vi "Trilateration.vi"(8 "direction":bool) -> (1 "new point z":dbl=0.11811869208701314, 2 "new point y":dbl=0.8159406539564933, 3 "new point x":dbl=0.4340593460435067)   [LabVIEW 2018]
doc: "Calculates position of a point in 3D space which is at known distances from three points."
uses:
  <vilib>/measure/NI_MAPro.lvlib
  <vilib>/measure/matone.llb/Extract Multiple Tone Information 1 Chan.vi
  <vilib>/Analysis/NI_AALBase.lvlib
  <vilib>/Analysis/3filter.llb/Butterworth Filter (DBL).vi
  <vilib>/Analysis/3filter.llb/Filter Passband Type.ctl
  <resource>/objmgr/daqmx.rc
  <vilib>/DAQmx/read.llb/DAQmx Read (Analog 2D DBL NChan NSamp).vi
  <vilib>/DAQmx/configure/timing.llb/DAQmx Timing (Sample Clock).vi
  <vilib>/DAQmx/create/channels.llb/DAQmx Create Channel (AI-Voltage-Basic).vi
  <vilib>/DAQmx/configure/trigger.llb/DAQmx Start Trigger (None).vi
panel:
  in  "physical channels":tag="Dev2/ai0:1"
  in  "Sampling rate":dbl=10000.0 format="%0.2f"
  in  "stop":bool
  out "Waveform Graph":dbl[][](graph)
  in  "Change":bool
  in  "sampling freq: fs":dbl=1.0 format="%0.2f"
  in  "z 3":dbl
  in  "y 3":dbl
  in  "x 3":dbl=1.0
  in  "z 2":dbl
  in  "y 2":dbl
  in  "x 2":dbl=1.0
  in  "z":dbl
  in  "y":dbl
  in  "x":dbl=1.0
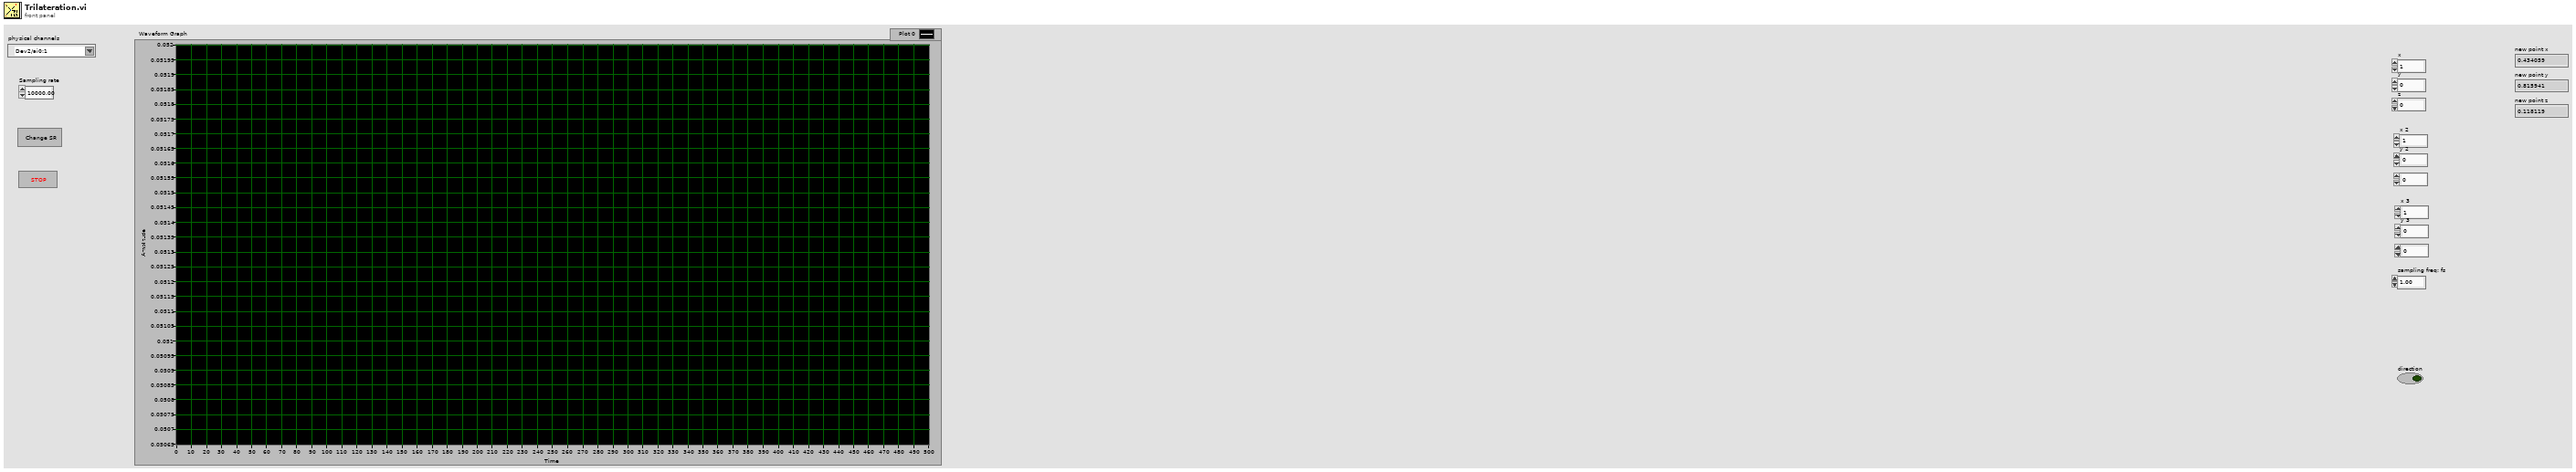
[diagram p1: front panel]
types:
  T1 = typedef "NI_AALBase.lvlib/Filter Passband Type.ctl" = enum32{"Lowpass", "Highpass", "Bandpass", "Bandstop"}
  T2 = cluster{"detected frequency":dbl, "detected amplitude":dbl, "detected phase (deg)":dbl}[]
  T3 = cluster{"[0]":cluster{"detected frequency":dbl, "detected amplitude":dbl, "detected phase (deg)":dbl}, "[1]":cluster{"detected frequency":dbl, "detected amplitude":dbl, "detected phase (deg)":dbl}, "[2]":cluster{"detected frequency":dbl, "detected amplitude":dbl, "detected phase (deg)":dbl}, "[3]":cluster{"detected frequency":dbl, "detected amplitude":dbl, "detected phase (deg)":dbl}, "[4]":cluster{"detected frequency":dbl, "detected amplitude":dbl, "detected phase (deg)":dbl}, "[5]":cluster{"detected frequency":dbl, "detected amplitude":dbl, "detected phase (deg)":dbl}, "[6]":cluster{"detected frequency":dbl, "detected amplitude":dbl, "detected phase (deg)":dbl}, "[7]":cluster{"detected frequency":dbl, "detected amplitude":dbl, "detected phase (deg)":dbl}, "[8]":cluster{"detected frequency":dbl, "detected amplitude":dbl, "detected phase (deg)":dbl}}
  T4 = cluster{"detected frequency":dbl, "detected amplitude":dbl, "detected phase (deg)":dbl}
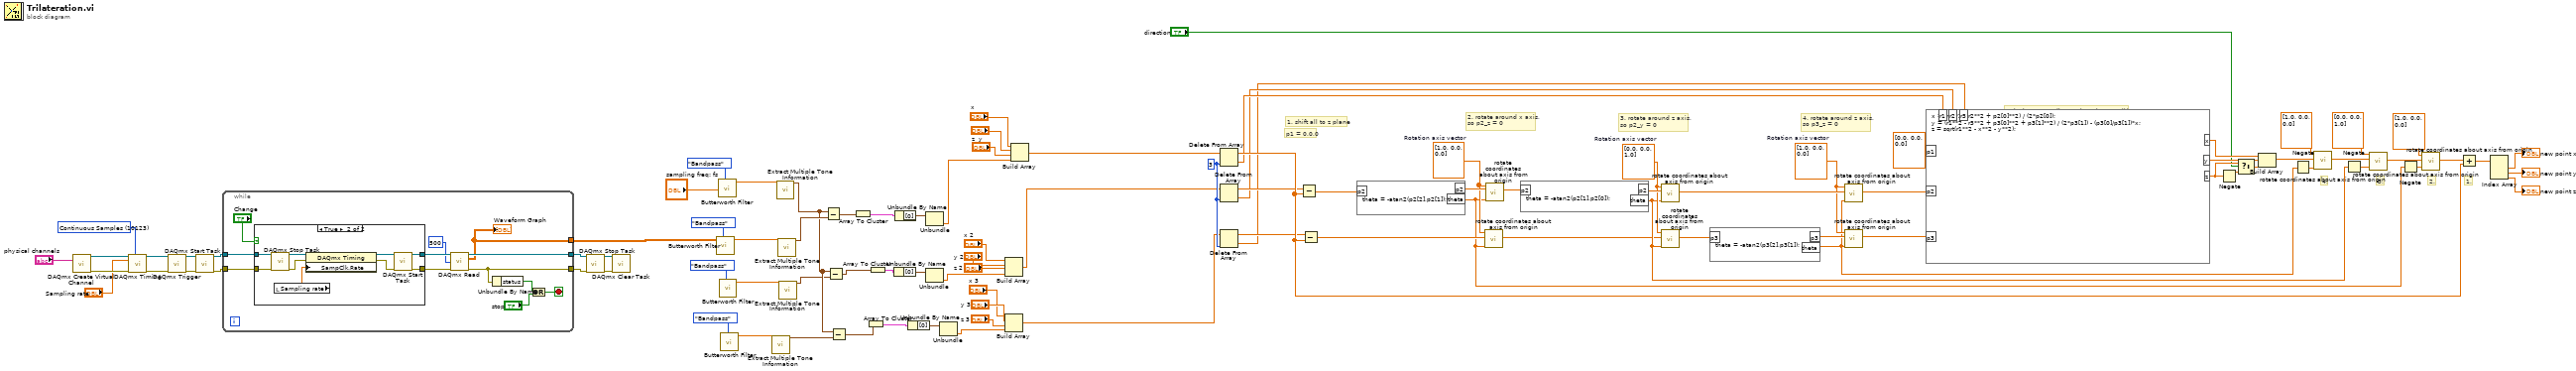
[diagram p0: block diagram]
diagram:
  w9 = 10123 items=["Finite Samples"=10178, "Continuous Samples"=10123, "Hardware Timed Single Point"=12522] ("sample mode")
  w65 = 3 ("index")
  w77 = dbl[] [1.0, 0.0, 0.0]  # Rotation axis vector
  w85 = dbl[] [1.0, 0.0, 0.0]  # Rotation axis vector
  w97 = dbl[] [0.0, 0.0, 1.0]  # Rotation axis vector
  # "1."
  # "2."
  # "3."
  # "4."
  # "Calculate, according to the rules on wiki"
  # "4. rotate around z axis,\nso p3_z = 0"
  # "2. rotate around x axis,\nso p2_z = 0"
  # "1. shift all to z plane"
  # "3. rotate around z axis,\nso p2_y = 0"
  # "p1 = 0,0,0"
  n1 = call-poly <vilib>:"DAQmx Create Virtual Channel.vi"("physical channels"="physical channels") -> ("task out"=w14:refnum<k21>, "error out"=w12:errorcluster)  [unwired: 13 in]
  n2 = call-poly <vilib>:"DAQmx Timing.vi"("task/channels in"=w14, "sample mode"=w9, "rate"="Sampling rate", "error in"=w12) -> ("task out"=w5:refnum<k21>, "error out"=w3:errorcluster)  [unwired: 10 in]
  n3 = call-poly <vilib>:"DAQmx Trigger.vi"("task/channels in"=w5, "error in"=w3) -> ("task out"=w4:refnum<k21>, "error out"=w2:errorcluster)  [unwired: 12 in]
  n4 = call <vilib>:"DAQmx Start Task.vi"("task/channels in"=w4, "error in"=w2) -> ("task out"=w7:refnum<k21>, "error out"=w8:errorcluster)  [unwired: 12 in]
  n5 = while {
    tunnel: w7 -> [w105]
    tunnel: [w110] -> w13
    tunnel: w8 -> [w103]
    tunnel: [w108] -> w11
    tunnel: [w99] -> w1
    stop <- w109 stop-if-true
    n6 = case shown="True" "Change" {
      tunnel: w105 -> [w112 w120]
      tunnel: [w112 w115] -> w104
      tunnel: w103 -> [w111 w119]
      tunnel: [w111 w113] -> w102
      frame False {
      }
      frame True {
        n7 = call <vilib>:"DAQmx Stop Task.vi"("task/channels in"=w120, "error in"=w119) -> ("task out"=w118:refnum<k21>, "error out"=w117:errorcluster)  [unwired: 12 in]
        n8 = local read "Sampling rate"() -> (w121:dbl)
        n9 = property class="DAQmx Timing"(reference=w118, error in=w117, "SampClk.Rate"=w121) -> (reference out=w116:refnum<k21>, error out=w114:errorcluster)
        n10 = call <vilib>:"DAQmx Start Task.vi"("task/channels in"=w116, "error in"=w114) -> ("task out"=w115:refnum<k21>, "error out"=w113:errorcluster)  [unwired: 12 in]
      }
    }
    n11 = call-poly <vilib>:"DAQmx Read.vi"("task/channels in"=w104, "number of samples per channel"=500, "error in"=w102) -> ("task out"=w110:refnum<k21>, "data"=w99:dbl[][], "error out"=w108:errorcluster)  [unwired: 10 in]
    "Waveform Graph" <- w99
    n12 = Unbundle By Name(w108) -> ("status"=w107:bool)
    n13 = Or(x=w107, y="stop") -> (x .or. y?=w109:bool)
  }
  n14 = call <vilib>:"DAQmx Stop Task.vi"("task/channels in"=w13, "error in"=w11) -> ("task out"=w16:refnum<k21>, "error out"=w15:errorcluster)  [unwired: 12 in]
  n15 = call <vilib>:"DAQmx Clear Task.vi"("task in"=w16, "error in"=w15) -> ()  [unwired: 13 in, 1 out]
  n16 = call-poly <vilib>:"Butterworth Filter.vi"("filter type"=Filter_Passband_Type."Bandpass", "X"=w1) -> ("Filtered X"=w44:dbl[])  [unwired: 6 in, 1 out]
  n17 = call-poly <vilib>:"Butterworth Filter.vi"("filter type"=Filter_Passband_Type."Bandpass", "sampling freq: fs"="sampling freq: fs") -> ("Filtered X"=w45:dbl[])  [unwired: 6 in, 1 out]
  n18 = call-poly <vilib>:"Butterworth Filter.vi"("filter type"=Filter_Passband_Type."Bandpass") -> ("Filtered X"=w43:dbl[])  [unwired: 7 in, 1 out]
  n19 = call-poly <vilib>:"Butterworth Filter.vi"("filter type"=Filter_Passband_Type."Bandpass") -> ("Filtered X"=w42:dbl[])  [unwired: 7 in, 1 out]
  n20 = call-poly <vilib>:"Extract Multiple Tone Information.vi"("time signal in"=w42) -> ("multiple tone information"=w51:T2)  [unwired: 12 in, 2 out]
  n21 = call-poly <vilib>:"Extract Multiple Tone Information.vi"("time signal in"=w45) -> ("multiple tone information"=w52:T2)  [unwired: 12 in, 2 out]
  n22 = call-poly <vilib>:"Extract Multiple Tone Information.vi"("time signal in"=w44) -> ("multiple tone information"=w53:T2)  [unwired: 12 in, 2 out]
  n23 = call-poly <vilib>:"Extract Multiple Tone Information.vi"("time signal in"=w43) -> ("multiple tone information"=w50:T2)  [unwired: 12 in, 2 out]
  n24 = Subtract(x=w52, y=w53) -> (x-y=w40:T2)
  n25 = Subtract(x=w52, y=w50) -> (x-y=w31:T2)
  n26 = Subtract(x=w52, y=w51) -> (x-y=w32:T2)
  n27 = Array To Cluster(array=w40) -> (cluster=w39:T3)
  n28 = Array To Cluster(array=w32) -> (cluster=w34:T3)
  n29 = Array To Cluster(array=w31) -> (cluster=w36:T3)
  n30 = Unbundle By Name(w36) -> ("[0]"=w35:T4)
  n31 = Unbundle By Name(w39) -> ("[0]"=w38:T4)
  n32 = Unbundle By Name(w34) -> ("[0]"=w33:T4)
  n33 = Unbundle(w35) -> ("detected phase (deg)"=w30:dbl)  [unwired: 2 out]
  n34 = Unbundle(w38) -> ("detected phase (deg)"=w37:dbl)  [unwired: 2 out]
  n35 = Unbundle(w33) -> ("detected phase (deg)"=w25:dbl)  [unwired: 2 out]
  n36 = Build Array("x 2", "y 2", "z 2", w30) -> (w26:dbl[])
  n37 = Build Array("x 3", "y 3", "z 3", w25) -> (w21:dbl[])
  n38 = Build Array("x", "y", "z", w37) -> (w41:dbl[])
  n39 = Delete From Array(array=w41, index=w65) -> (deleted portion=w61:dbl, array with subset deleted=w64:dbl[])  [unwired: 1 in]
  n40 = Delete From Array(array=w26, index=w65) -> (deleted portion=w60:dbl, array with subset deleted=w63:dbl[])  [unwired: 1 in]
  n41 = Delete From Array(array=w21, index=w65) -> (deleted portion=w59:dbl, array with subset deleted=w62:dbl[])  [unwired: 1 in]
  n42 = Subtract(x=w63, y=w64) -> (x-y=w87:dbl[])
  n43 = Subtract(x=w62, y=w64) -> (x-y=w86:dbl[])
  n44 = formula code="theta = -atan2(p2[2],p2[1]);"("p2"=w87) -> ("theta"=w75:dbl, "p2"=w88:dbl[])
  n45 = call "rotate coordinates about axis from origin.vi"("Angle (CCW)"=w75, "Point to rotate"=w86, "Rotation axis vector"=w85) -> ("New position"=w83:dbl[])  [unwired: 8 in]
  n46 = call "rotate coordinates about axis from origin.vi"("Angle (CCW)"=w75, "Point to rotate"=w88, "Rotation axis vector"=w85) -> ("New position"=w84:dbl[])  [unwired: 8 in]
  n47 = formula code="theta = -atan2(p2[1],p2[0]);"("p2"=w84) -> ("theta"=w92:dbl, "p2"=w98:dbl[])
  n48 = call "rotate coordinates about axis from origin.vi"("Angle (CCW)"=w92, "Point to rotate"=w98, "Rotation axis vector"=w97) -> ("New position"=w79:dbl[])  [unwired: 8 in]
  n49 = call "rotate coordinates about axis from origin.vi"("Angle (CCW)"=w92, "Point to rotate"=w83, "Rotation axis vector"=w97) -> ("New position"=w82:dbl[])  [unwired: 8 in]
  n50 = formula code="theta = -atan2(p3[2],p3[1]);"("p3"=w82) -> ("theta"=w71:dbl, "p3"=w81:dbl[])
  n51 = call "rotate coordinates about axis from origin.vi"("Angle (CCW)"=w71, "Point to rotate"=w79, "Rotation axis vector"=w77) -> ("New position"=w78:dbl[])  [unwired: 8 in]
  n52 = call "rotate coordinates about axis from origin.vi"("Angle (CCW)"=w71, "Point to rotate"=w81, "Rotation axis vector"=w77) -> ("New position"=w80:dbl[])  [unwired: 8 in]
  n53 = formula code="x = (r1**2 - r2**2 + p2[0]**2) / (2*p2[0]);\ny = (r1**2 - r3**2 + p3[0]**2 + p3[1]**2) / (2*p3[1]) - (p3[0]/p3[1])*x;\nz = sqrt(r1**2 - x**2 - y**2);"("p1"=dbl[] [0.0, 0.0, 0.0] ("input variable"), "p2"=w78, "p3"=w80, "r1"=w61, "r2"=w60, "r3"=w59) -> ("x"=w95:dbl, "y"=w94:dbl, "z"=w90:dbl)
  n54 = Negate(x=w90) -> (-x=w91:dbl)
  n55 = Select(t=w90, s="direction", f=w91) -> (s? t:f=w89:dbl)
  n56 = Build Array(w95, w94, w89) -> (w73:dbl[])
  n57 = Negate(x=w71) -> (-x=w74:dbl)
  n58 = call "rotate coordinates about axis from origin.vi"("Angle (CCW)"=w74, "Point to rotate"=w73, "Rotation axis vector"=dbl[] [1.0, 0.0, 0.0]) -> ("New position"=w70:dbl[])  [unwired: 8 in]
  n59 = Negate(x=w92) -> (-x=w76:dbl)
  n60 = call "rotate coordinates about axis from origin.vi"("Angle (CCW)"=w76, "Point to rotate"=w70, "Rotation axis vector"=dbl[] [0.0, 0.0, 1.0]) -> ("New position"=w67:dbl[])  [unwired: 8 in]
  n61 = Negate(x=w75) -> (-x=w68:dbl)
  n62 = call "rotate coordinates about axis from origin.vi"("Angle (CCW)"=w68, "Point to rotate"=w67, "Rotation axis vector"=dbl[] [1.0, 0.0, 0.0]) -> ("New position"=w66:dbl[])  [unwired: 8 in]
  n63 = Add(x=w66, y=w64) -> (x+y=w57:dbl[])
  n64 = Index Array(array=w57) -> (element #1=→"new point x":dbl, element #2=→"new point y":dbl, element #3=→"new point z":dbl)  [unwired: 3 in]
